vi "Loop_ACT.vi"(10 "Camera Occurance":refnum<k4>) -> ()   [LabVIEW 2017, in "VisionHW.lvlib"]
uses:
  VisionHW.lvlib
  TypeDefs/CLUST_Targeting Data.ctl
  TypeDefs/CLUST_Cube Data.ctl
  TypeDefs/CLUST_Road Navigation Data.ctl
  TypeDefs/ENUM_Vision_Commands.ctl
  _SHARE ALL/Global Share All/Global_STOP.vi
  Globals/Global_Vision_CMDs.vi
  Globals/Global_Vision_Data.vi
panel:
  out "Targeting Data":T1
  out "Target Data":string
  in  "Vision Command":string
  out "Cycle Time (S)":dbl format="%.3g"
  in  "Target Time(ms)":u32=50
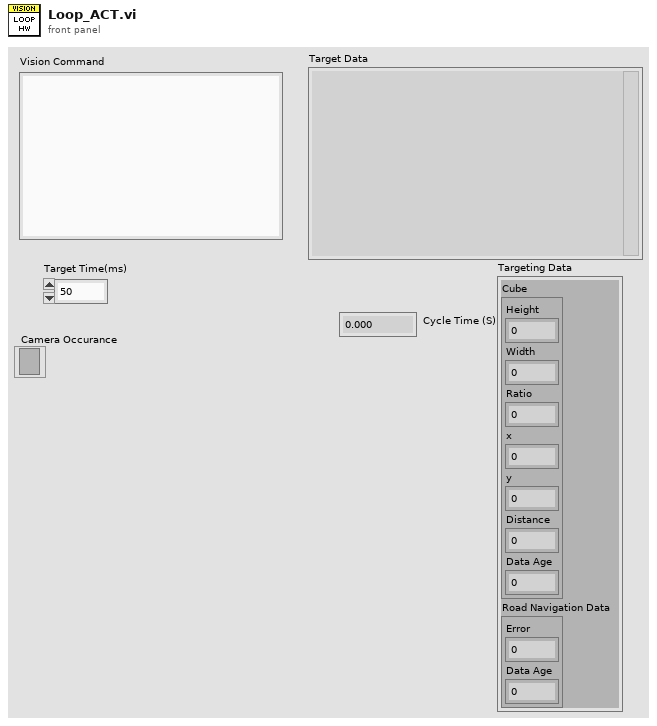
[diagram p1: front panel]
types:
  T1 = typedef "VisionHW.lvlib/CLUST_Targeting Data.ctl" = cluster{"Cube ":T2, "Road Navigation Data":T3}
  T2 = typedef "VisionHW.lvlib/CLUST_Cube Data.ctl" = cluster{"Height":dbl, "Width":dbl, "Ratio":dbl, "x":i32, "y":i32, "Distance ":i32, "Data Age":dbl}
  T3 = typedef "VisionHW.lvlib/CLUST_Road Navigation Data.ctl" = cluster{"Error":i32, "Data Age":dbl}
  T4 = typedef "ENUM_Vision_Commands.ctl" = enum16{"Init", "NoOp", "ResetCamera", "VideoOn", "VideoOff", "CubeDetection", "RoadNavigation"}
  T5 = typedef "WPI_SerialPortRef.ctl" = cluster{"DevStatus":errorcluster, "Serial Port Name":refnum<visa-resource-name>}
  T6 = cluster{"SerialRefOut":T5, " Log Output":string, "CMD":T4, "Target Time(ms)":u32, "Current Time":timestamp, "Previous Time":timestamp, "Cycle Time (S)":dbl, "Targeting Data":T1}
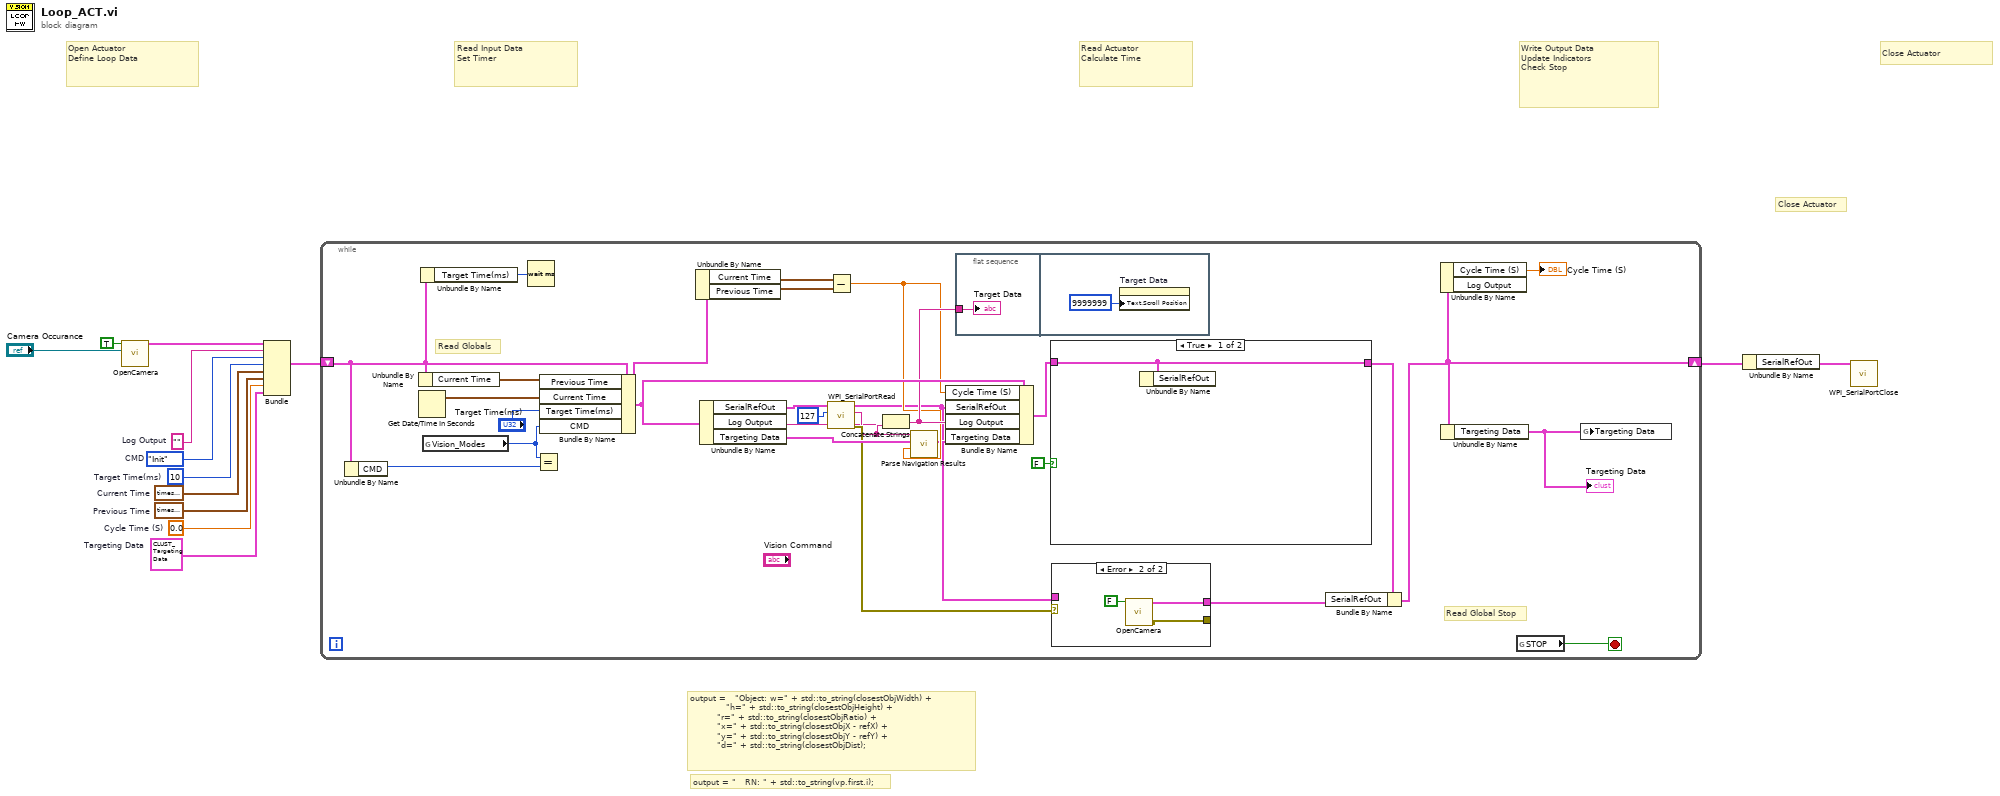
[diagram p0: block diagram]
diagram:
  w5 = T1 {"Cube "={"Height"=0.0, "Width"=0.0, "Ratio"=0.0, "x"=0, "y"=0, "Distance "=0, "Data Age"=0.0}, "Road Navigation Data"={"Error"=0, "Data Age"=0.0}}  # Targeting Data
  w8 = ENUM_Vision_Commands."Init"  # CMD
  w6 = 0.0  # Cycle Time (S)
  w13 = timestamp(0 s since 1904-01-01)  # Previous Time
  w12 = timestamp(0 s since 1904-01-01)  # Current Time
  w11 = u32 10  # Target Time(ms)
  w10 = ""  # Log Output
  # "output = \"   RN: \" + std::to_string(vp.first.i);"
  # "output =   \"Object: w=\" + std::to_string(closestObjWidth) +\n\t\t   \t\t\t\t\t  \"h=\" + std::to_string(closestObjHeight) +\n\t\t\t\t\t\t\t  \"r=\" + std::to_string(closestObjRatio) +\n\t\t\t\t\t\t\t  \"x=\" + std::to_string(closestObjX - refX) +\n\t\t\t\t\t\t\t  \"y=\" + std::to_string(closestObjY - refY) +\n\t\t\t\t\t\t\t  \"d=\" + std::to_string(closestObjDist);"
  # "Close Actuator"
  # "Write Output Data\nUpdate Indicators\nCheck Stop"
  # "Read Actuator\nCalculate Time"
  # "Read Input Data\nSet Timer"
  # "Open Actuator\nDefine Loop Data"
  # "Close Actuator"
  n1 = call "OpenCamera.vi"("Camera Occurance"="Camera Occurance", "Wait For Occurance"=TRUE) -> ("SerialRefOut"=w7:T5)  [unwired: 8 in, 1 out]
  n2 = Bundle("SerialRefOut"=w7, "Log Output"=w10, "CMD"=w8, "Target Time(ms)"=w11, "Current Time"=w12, "Previous Time"=w13, "Cycle Time (S)"=w6, "Targeting Data"=w5) -> (w4:T6)  [unwired: 1 in]
  n3 = while {
    shift-right: [w17] -> w9
    shift-left: w4 -> [w31]
    stop <- w41 stop-if-true
    # "Read Globals"
    # "Read Global Stop"
    n4 = Unbundle By Name(w31) -> ("CMD"=w30:T4)
    n5 = Unbundle By Name(w31) -> ("Current Time"=w39:timestamp)
    n6 = Get Date/Time In Seconds() -> (seconds since 1Jan1904=w40:timestamp)
    n7 = Unbundle By Name(w31) -> ("Target Time(ms)"=w34:u32)
    n8 = global read "Global_Vision_CMDs.vi" "Vision_Modes"() -> (w32:T4)
    n9 = Wait (ms)(milliseconds to wait=w34) -> ()  [unwired: 1 out]
    n10 = Equal?(x=w32, y=w30) -> ()  [unwired: 1 out]
    n11 = Bundle By Name(cluster=w31, "Previous Time"=w39, "Current Time"=w40, "Target Time(ms)"="Target Time(ms)", "CMD"=w32) -> (w35:T6)
    n12 = Unbundle By Name(w35) -> ("Current Time"=w38:timestamp, "Previous Time"=w37:timestamp)
    n13 = Unbundle By Name(w35) -> ("SerialRefOut"=w27:T5, "Log Output"=w14:string, "Targeting Data"=w23:T1)
    n14 = Subtract(x=w38, y=w37) -> (x-y=w24:dbl)
    n15 = call <vilib>:"WPI_SerialPortRead.vi"("Num Bytes to Read"=u32 127 ("byte count"), "SerialPortRef"=w27) -> ("error out"=w20:errorcluster, "Buffer"=w15:string, "SerialPortRef"=w16:T5)  [unwired: 7 in]
    n16 = Concatenate Strings(w14, w15) -> (w29:string)
    n17 = call "Parse Navigation Results.vi"("Cycle Time"=w24, "Targeting Data In"=w23, "Target Data"=w15) -> ("Targeting Data Out"=w22:T1)  [unwired: 8 in]
    n18 = Bundle By Name(cluster=w35, "Cycle Time (S)"=w24, "SerialRefOut"=w16, "Log Output"=w29, "Targeting Data"=w22) -> (w26:T6)
    n19 = flat-sequence {
      tunnel: w29 -> [w46]
      frame #0 {
        "Target Data" <- w46
      }
      frame #1 {
        n20 = property on="Target Data" class="Str"("Text.Scroll Position"=u32 9999999) -> ()  [unwired: 2 in, 2 out]
      }
    }
    n21 = case shown="True" FALSE {
      tunnel: w26 -> [w48 w49]
      tunnel: [w48 w49] -> w19
      frame True {
        n22 = Unbundle By Name(w48) -> ()  [unwired: 1 out]
      }
      frame False {
      }
    }
    n23 = case shown="Error" w20 {
      tunnel: [_ w44] -> _
      tunnel: [w42 w43] -> w18
      tunnel: w16 -> [w42 _]
      frame No Error {
      }
      frame Error {
        n24 = call "OpenCamera.vi"("Wait For Occurance"=FALSE) -> ("error out"=w44:errorcluster, "SerialRefOut"=w43:T5)  [unwired: 9 in]
      }
    }
    n25 = Bundle By Name(cluster=w19, "SerialRefOut"=w18) -> (w17:T6)
    n26 = Unbundle By Name(w17) -> ("Cycle Time (S)"=→"Cycle Time (S)":dbl)  [unwired: 1 out]
    n27 = Unbundle By Name(w17) -> ("Targeting Data"=w21:T1)
    "Targeting Data" <- w21
    n28 = global read "Global_STOP.vi" "STOP"() -> (w41:bool)
    n29 = global write "Global_Vision_Data.vi" "Targeting Data"(w21) -> ()
  }
  n30 = Unbundle By Name(w9) -> ("SerialRefOut"=w3:T5)
  n31 = call <vilib>:"WPI_SerialPortClose.vi"("SerialPortRef"=w3) -> ()  [unwired: 10 in, 1 out]
